vi "Global.vi"() -> ()   [LabVIEW 2014]
uses:
  Others/Control cluster.ctl
  <vilib>/LVH/AR Drone Toolkit/Decode NavData/Typedefs/NavData Demo.ctl
  <vilib>/LVH/AR Drone Toolkit/AR Drone.lvlib
panel:
  out "Refresh rate Video Acquisition":i64
  out "Reset OCR":bool
  in  "Land/takeOff":bool=TRUE
  in  "Adjustments":cluster{"Sensitivity":dbl, "Null Zone":dbl}={"Sensitivity"=1.0, "Null Zone"=1.0} {"Null Zone" scale=0.0..5.0; "Sensitivity" scale=0.0..5.0}
  out "Optical Flow Video Stream":T1(plugin-control)
  out "Rectangle":T2
  out "Gray IMAQ":T1(plugin-control)
  in  "stop":bool=TRUE
  out "Control Cluster 2":T3 {"Yaw Speed" scale=-1.0..1.0; "Vertical Speed" scale=-1.0..1.0; "Pitch" scale=-1.0..1.0; "Roll" scale=-1.0..1.0}
  out "Hover":bool
  out "NavData Out 2":T4={"control state"=enum."TRANS_LANDING", "battery percentage"=75, "pitch (deg)"=0.053, "roll (deg)"=0.137, "yaw (deg)"=115.875, "altitude (cm)"=0, "vx (cm/s)?"=0.0, "vy (cm/s)?"=0.0, "vz (cm/s)?"=0.0, "detection cam type"=3}
  out "Control Cluster":T3={"Roll"=-0.03, "Pitch"=-0.052222222, "Vertical Speed"=0.0, "Yaw Speed"=0.0} {"Yaw Speed" scale=-1.0..1.0; "Vertical Speed" scale=-1.0..1.0; "Pitch" scale=-1.0..1.0; "Roll" scale=-1.0..1.0}
  out "B&W IMAQ with rectangle":T1(plugin-control)
  out "Raw video":picture
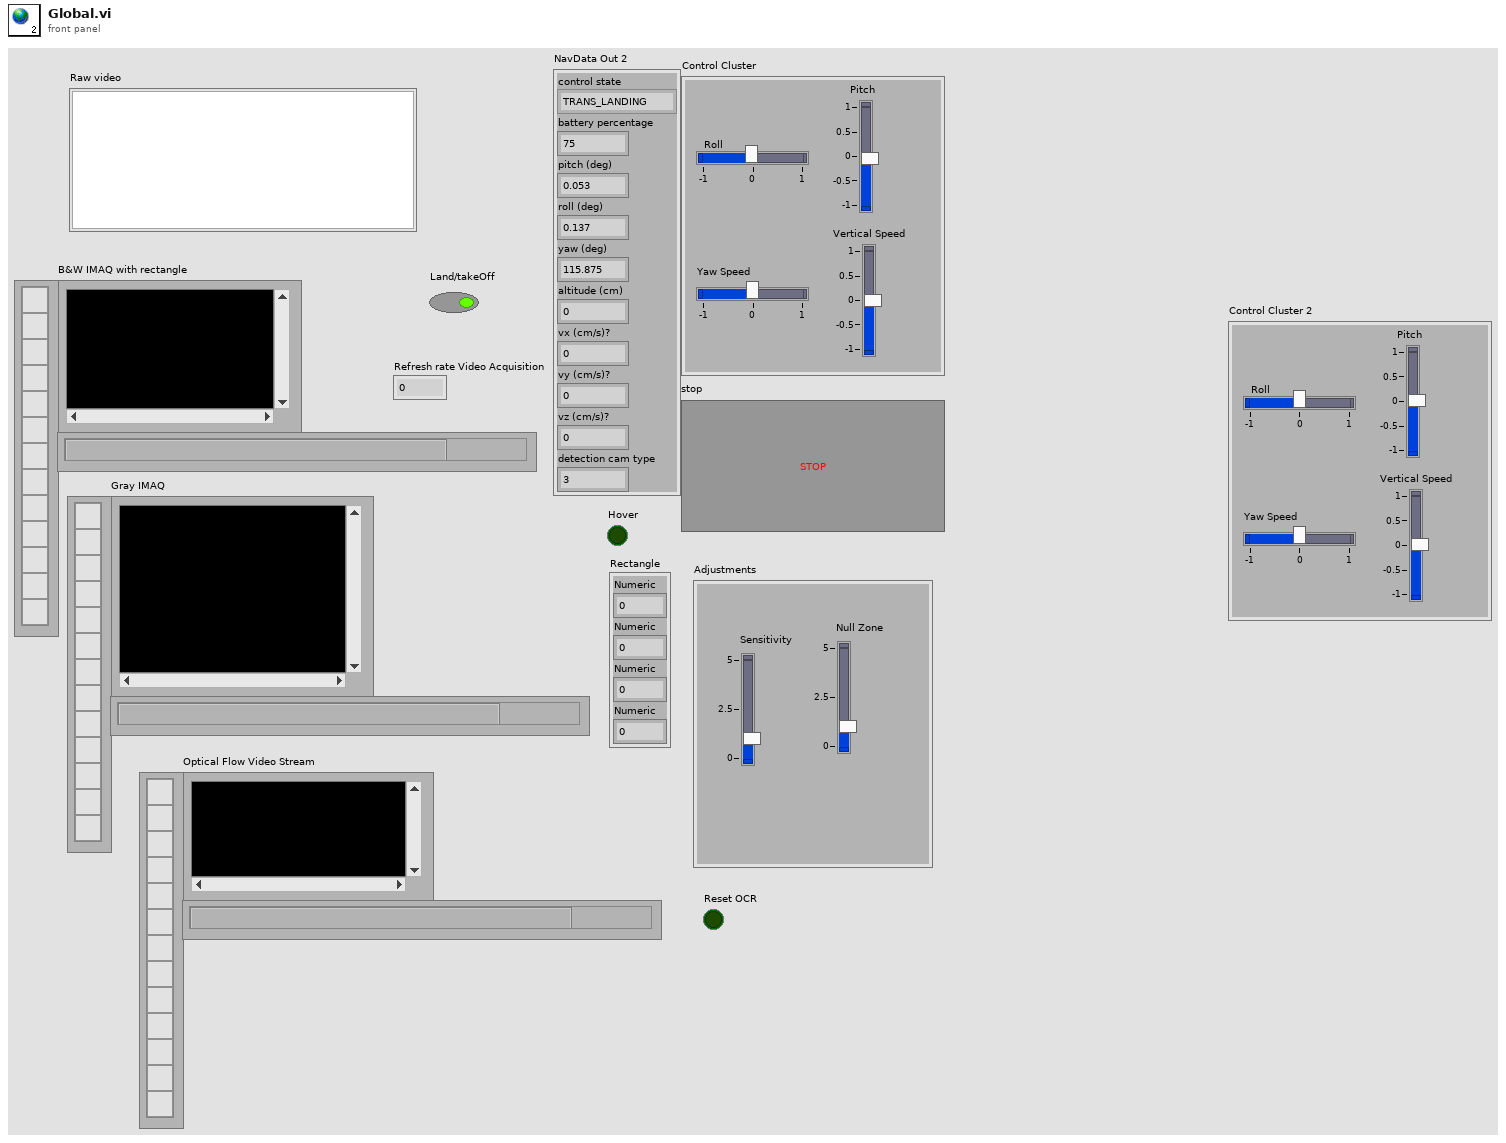
[diagram p1: front panel]
types:
  T1 = typedef "IMAQ Image.ctl" = refnum<image>
  T2 = cluster{"Numeric":dbl, "Numeric":dbl, "Numeric":dbl, "Numeric":dbl}
  T3 = typedef "Control cluster.ctl" = cluster{"Roll":sgl, "Pitch":sgl, "Vertical Speed":sgl, "Yaw Speed":sgl}
  T4 = typedef "AR Drone.lvlib/NavData Demo.ctl" = cluster{"control state":enum32{"DEFAULT", "INIT", "LANDING", "FLYING", "HOVERING", "TEST", "TRANS_TAKEOFF", "TRANS_GOTOFIX", "TRANS_LANDING"}, "battery percentage":u32, "pitch (deg)":sgl, "roll (deg)":sgl, "yaw (deg)":sgl, "altitude (cm)":u32, "vx (cm/s)?":sgl, "vy (cm/s)?":sgl, "vz (cm/s)?":sgl, "detection cam type":u32}
diagram:
